vi "Load.vi"(8 "error in (no error)":errorcluster, 10 "Path":path) -> (0 "error out":errorcluster, 3 "LVProject out":refnum<class "LVProject.lvclass">)   [LabVIEW 2020, in "GPack.lvlib" / "LVProject.lvclass"]
uses:
  LVProject.lvclass
  LVProject.lvclass/LVProject.ctl
  <vilib>/xml/Load XML File.vi
  <vilib>/xml/NI_XML.lvlib
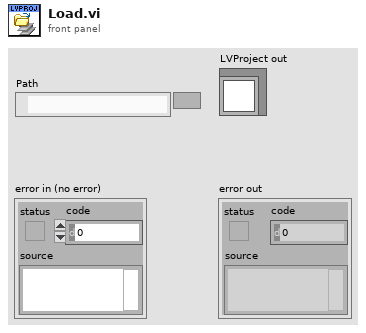
[diagram p1: front panel]
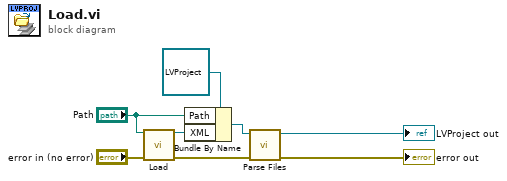
[diagram p0: block diagram]
diagram:
  n1 = call-poly <vilib>:"Load.vi"("path to XML document"="Path", "error in (no error)"="error in (no error)") -> ("DOM document out"=w4:refnum<k20>, "error out"=w2:errorcluster)  [unwired: 11 in, 1 out]
  n2 = Bundle By Name(cluster=refnum<class "LVProject.lvclass"> refnum ("LVProject in"), "Path"="Path", "XML"=w4) -> (w7:refnum<class "LVProject.lvclass">)
  n3 = call "Parse Files.vi"("error in (no error)"=w2, "LVProject in"=w7) -> ("error out"=→"error out":errorcluster, "LVProject out"=→"LVProject out":refnum<class "LVProject.lvclass">)  [unwired: 8 in]
